vi "uA_Measurement_kit_v2.vi"() -> ()   [LabVIEW 2015]
uses:
  Range_Shunt_selector.ctl
  <vilib>/Waveform/WDTFileIO.llb/ Write Waveform to File.vi
  <vilib>/Waveform/WDTFileIO.llb/Read Waveform from File.vi
  <vilib>/Utility/config.llb/Write Key (I32).vi
  <vilib>/Utility/config.llb/Write Key (Boolean).vi
  <vilib>/Utility/config.llb/Read Key (I32).vi
  <vilib>/Utility/config.llb/Read Key (Boolean).vi
  <vilib>/measure/madcrms.llb/Basic Averaged DC-RMS for 1 Chan.vi
  <resource>/objmgr/daqmx.rc
  <vilib>/Utility/config.llb/NI_LVConfig.lvlib
  <vilib>/measure/NI_MAPro.lvlib
panel:
  out "error out 3":errorcluster
  out "PhysicalChanName":tag
  out "DEV SN":u64 format="%.0x"
  out "mARange":dbl
  out "Boolean":bool
  out "DevSerialNum":u32
  in  "uA_bank0":dbl=1.5 format="%#_13g"
  out "Task out":refnum<k21>="Stop"
  out "Sample rate":dbl=20000.0 format="%#_13g"
  out "Clear":bool=TRUE
  out "Ver":string
  out "seconds since 1Jan1904":timestamp
  in  "Tab Control":enum32{"Current Tracking", "Logging"}(tab)
  out "out_range":bool
  in  "Save setting":bool
  out "PW_Source":bool
  out "EX_IN_INdicator":bool
  in  "LDO":string
  out "Lable.Unit_VOl_MA_UA":string
  in  "Ext PW Vol Monitor":bool
  out "POWER ON_OFF":bool
  out "vbat_lb":dbl format="%#_4f"
  in  "bypass Shunt":bool
  in  "Internal PW":bool
  in  "USB":tag="Dev1"
  out "schematic":bool
  in  "Save":bool
  in  "Load":bool
  out "uA_bank1":dbl
  in  "Calib":bool
  in  "Power ON/OFF":bool
  in  "Profile":enum16{"SAM", "DIANA", "Hi-POWER", "Other..."}(ring)
  in  "Take Picture":bool
  in  "Orginal":bool
  in  "Clear Graph":bool
  in  "ZOOM M1M2":bool
  in  "ZOOM -":bool
  in  "ZOOM +":bool
  in  "stop":bool
  out "Vbat":dbl format="%#.3f"
  in  "Measure":bool
  in  "Range - Shunts":T1
  out "PW_Internal_Source":dbl
  out "Min":dbl
  out "Max":dbl
  out "Delta(s)":sgl
  in  "Center":bool
  out "Avg":dbl
  out "Waveform_main":waveform(sgl)(graph)
  out "Waveform_sub":waveform(dbl)(graph)
  out "Average (uA)":dbl format="%#_6f"
  in  "Vout  - Vbat profile":enum16{"3.8VDC", "2.9VDC", "By Pass", "4.0VDC"}(ring)=enum."2.9VDC" caption="Vout  - Vbat"
  # "µPower kit V2.2"
  # "Vbat"
  # "Vdut- Vbat"
  # "DUT"
  # "Rs"
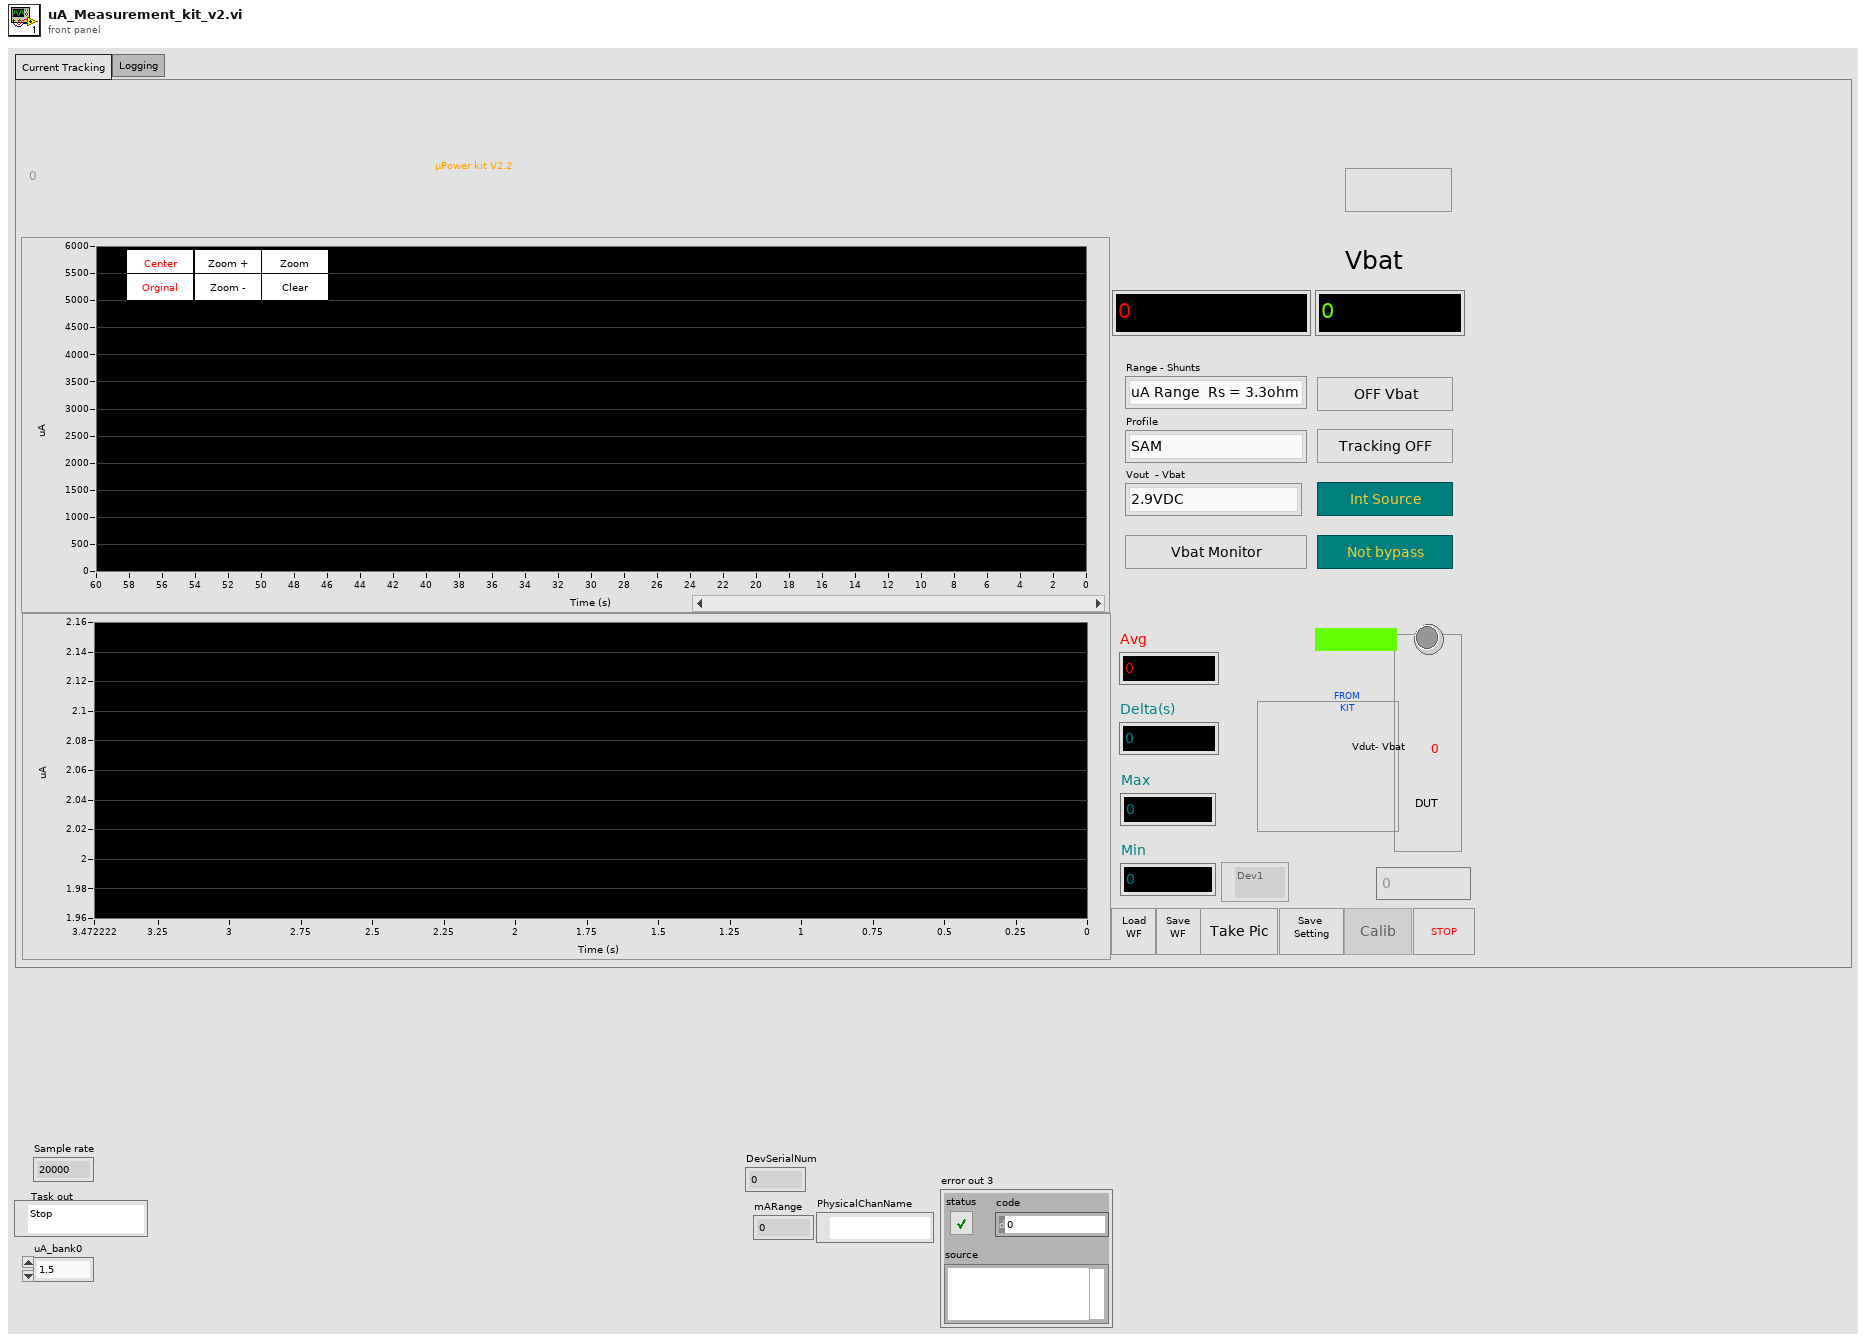
[diagram p1: front panel]
types:
  T1 = typedef "Range_Shunt_selector.ctl" = enum16{"uA Range  Rs = 3.3ohm", "mA Range Rs = 3.3ohm", "mA Range Rs = 1ohm", "mA Range Rs = 1ohm - X2"}
  T2 = enum8{"Enabled", "Disabled", "Disabled and Grayed Out"}
  T3 = typedef "NI_LVConfig.lvlib/Config Data RefNum.ctl" = refnum<k1>
  T4 = enum16{"Internal PW Source", "External PW Source"}
  T5 = enum16{"Turn On bypass - Off Shunt", "Turn Off bypass - On Shunt"}
  T6 = typedef "LVCursorListTypeDef.ctl" = cluster{"Name":string, "Color":u32, "Style":u8, "Point Style":u8, "Name Visible":bool, "Allow Drag":bool, "Cursor Mode":u32, "Plot":i32, "Index":i32, "Position":cluster{"X":dbl, "Y":dbl}, "X Scale":u32, "Y Scale":u32, "Watch Plots":i32[], "Watch All Plots":bool, "Plot Area":i32, "Label Offset":cluster{"X":dbl, "Y":dbl}}[]
  T7 = typedef "imagedata.ctl" = cluster{"image type":i32, "image depth":i32, "image":u8[], "mask":u8[], "colors":u32[], "Rectangle":cluster{"left":i16, "top":i16, "right":i16, "bottom":i16}}
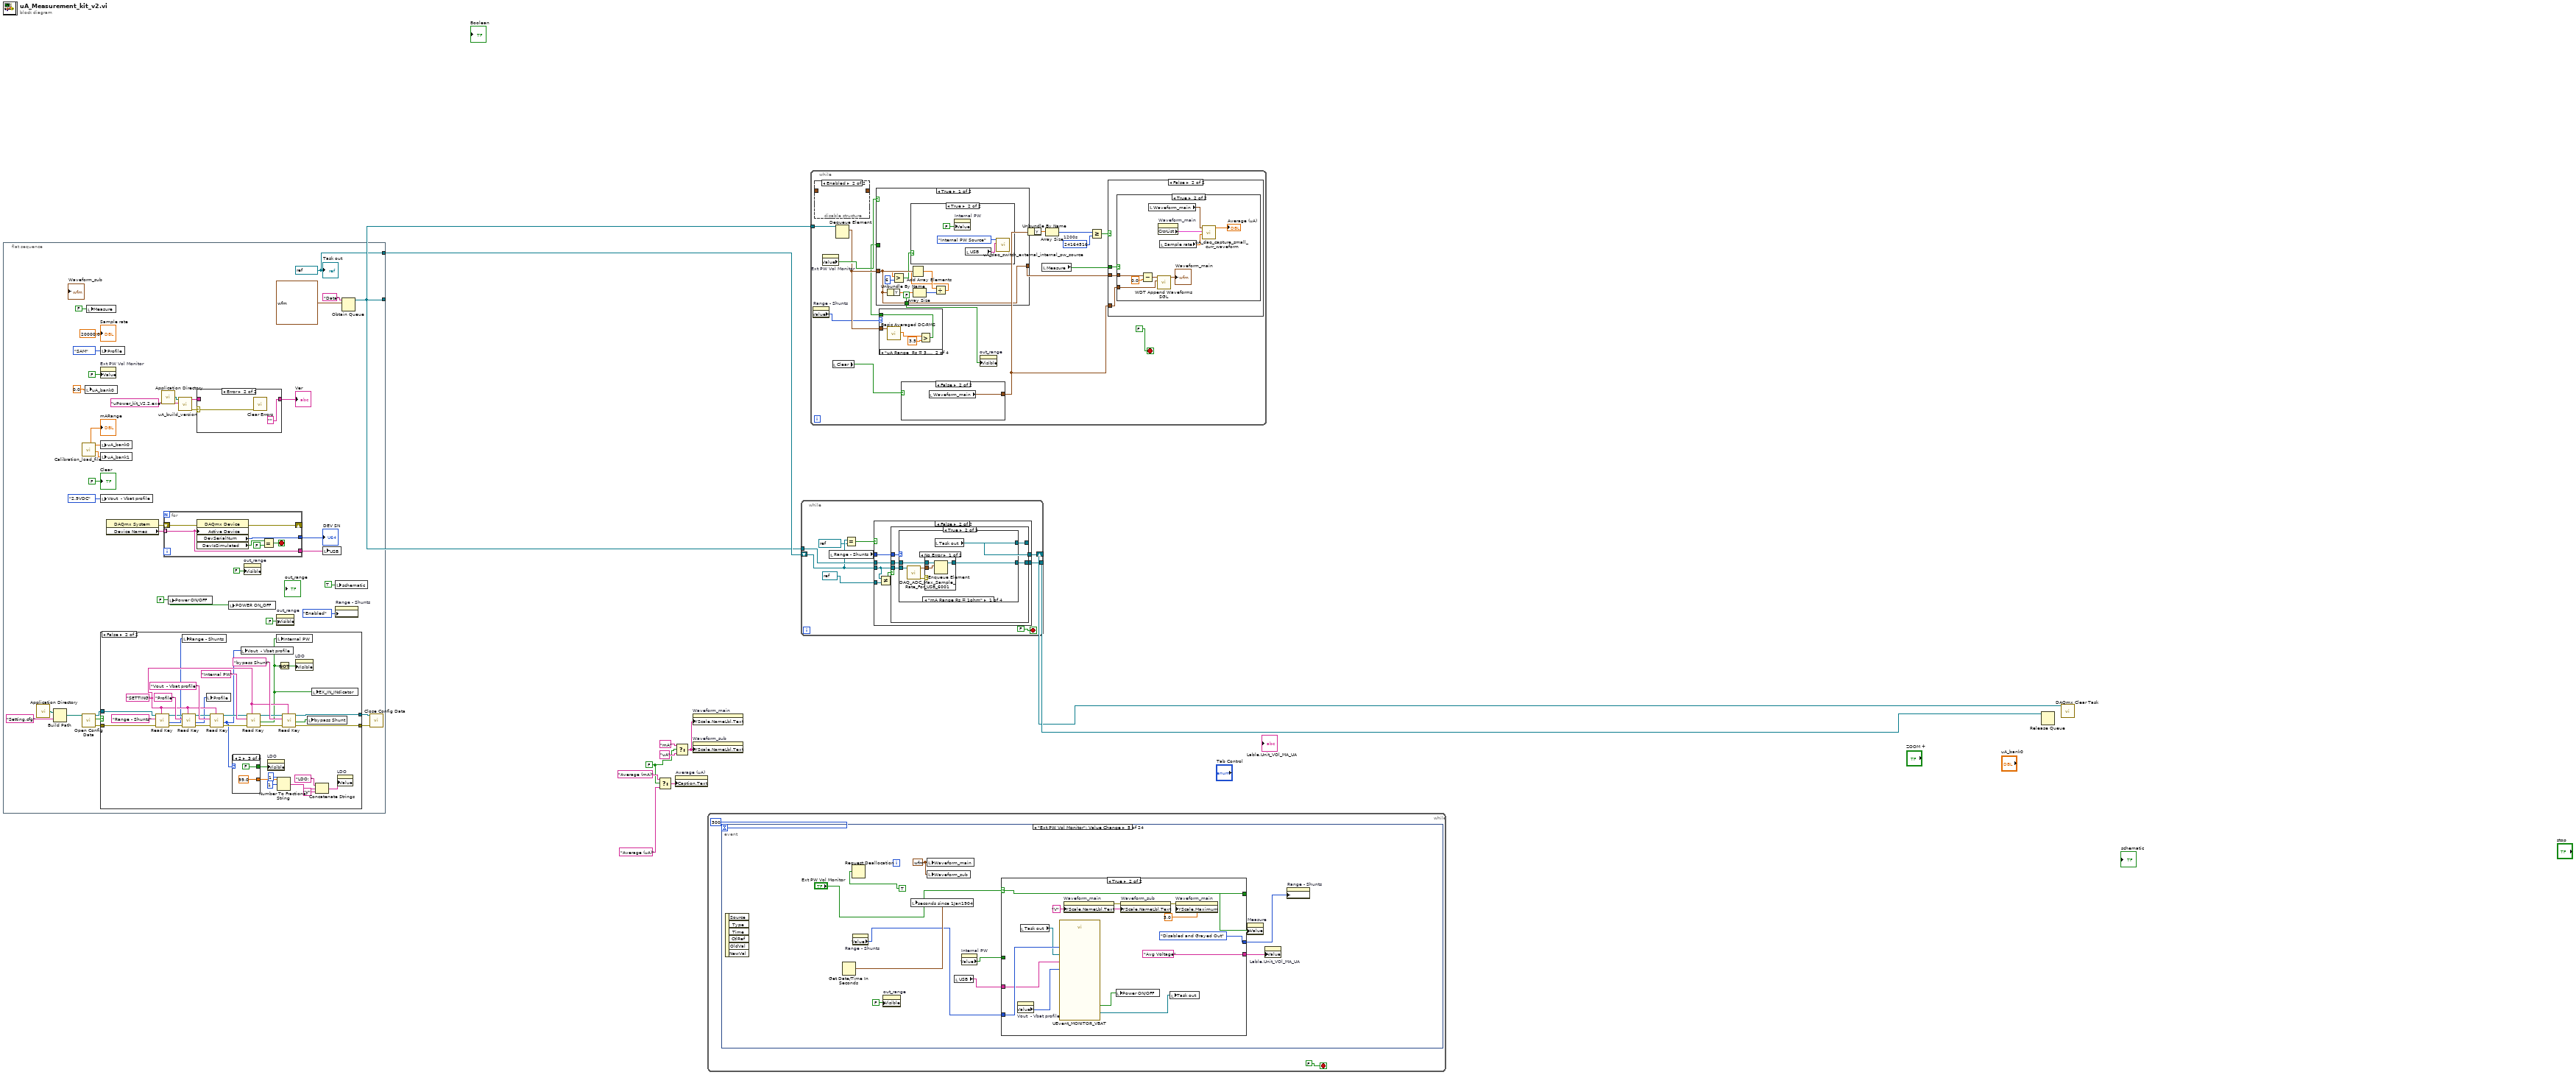
[diagram p0: block diagram]
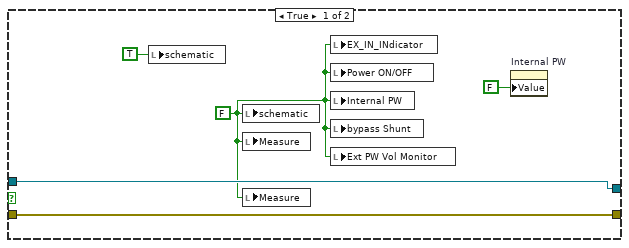
[diagram p2: hidden frame]
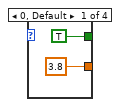
[diagram p3: hidden frame]
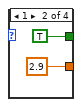
[diagram p4: hidden frame]
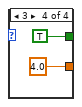
[diagram p5: hidden frame]
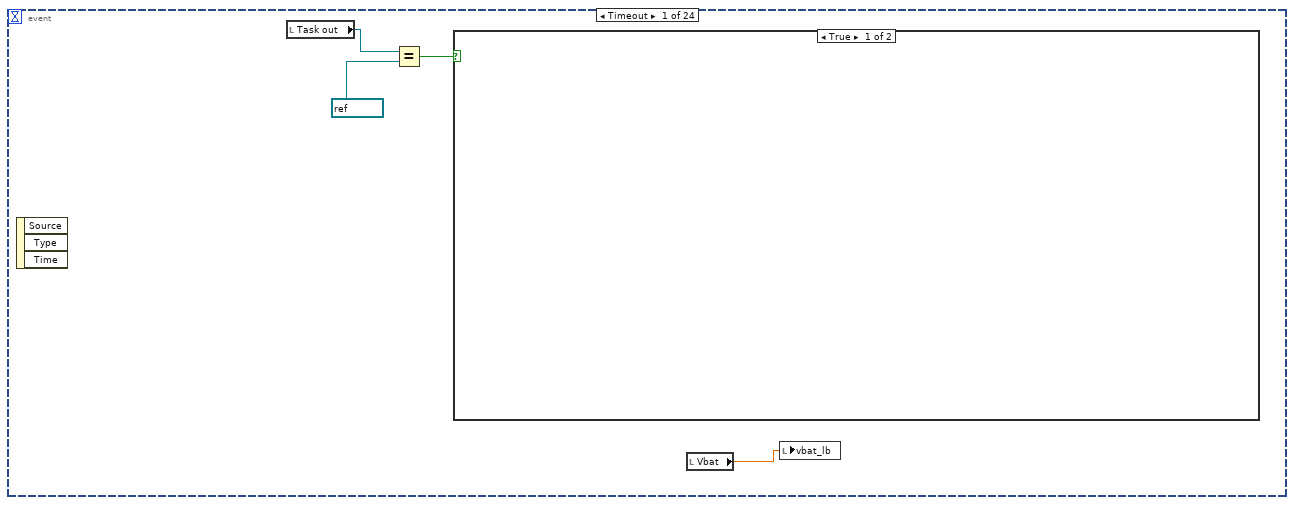
[diagram p7: hidden frame]
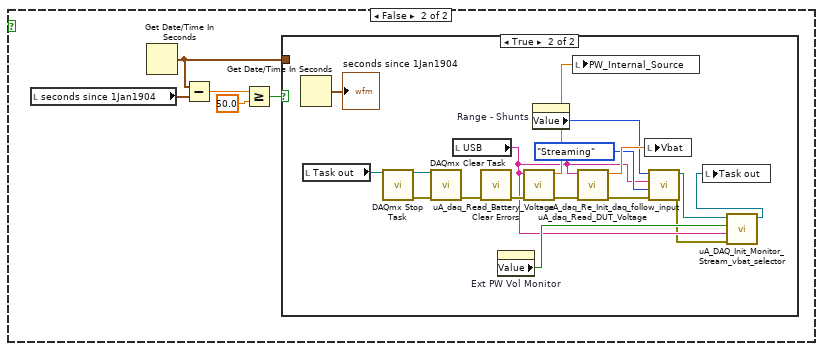
[diagram p8: hidden frame]
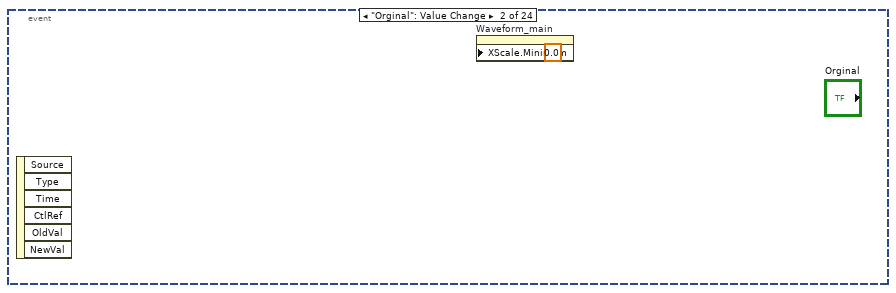
[diagram p10: hidden frame]
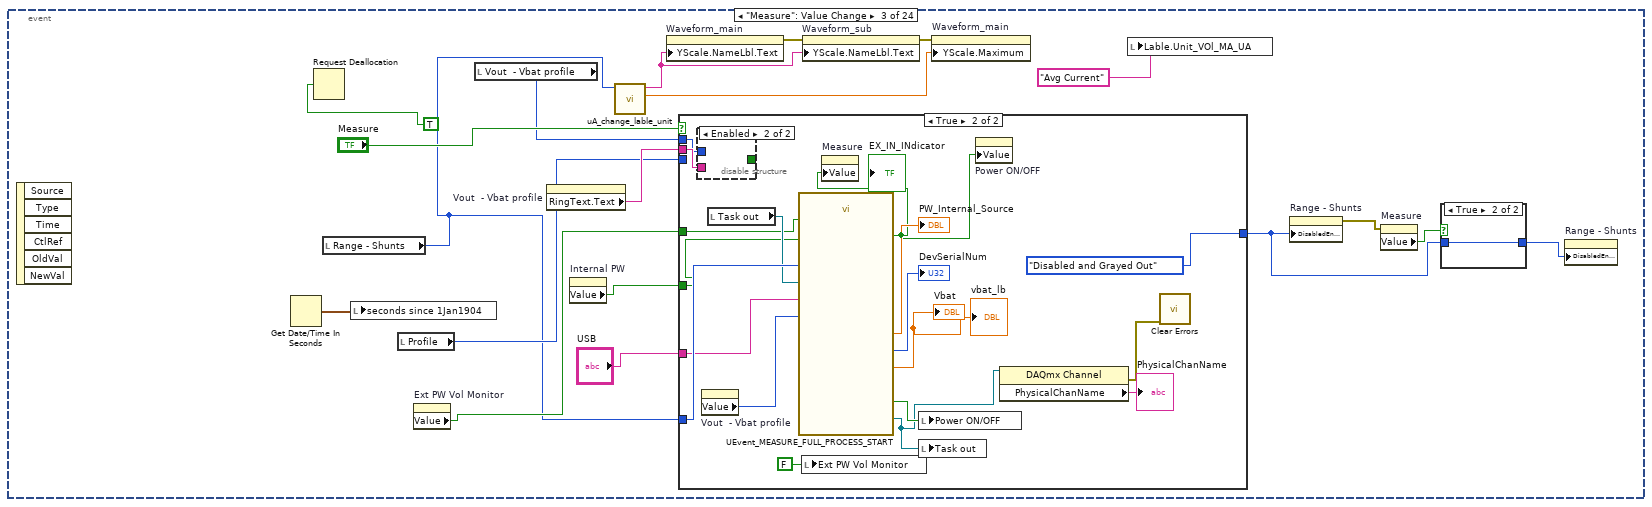
[diagram p11: hidden frame]
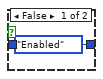
[diagram p12: hidden frame]
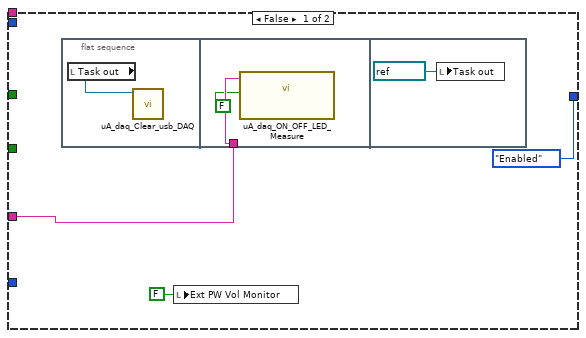
[diagram p13: hidden frame]
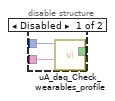
[diagram p14: hidden frame]
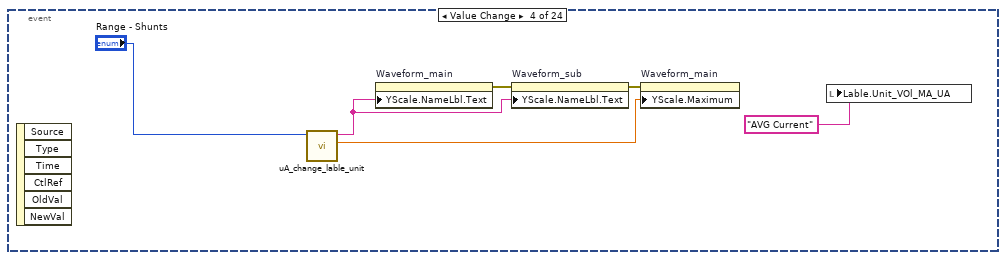
[diagram p15: hidden frame]
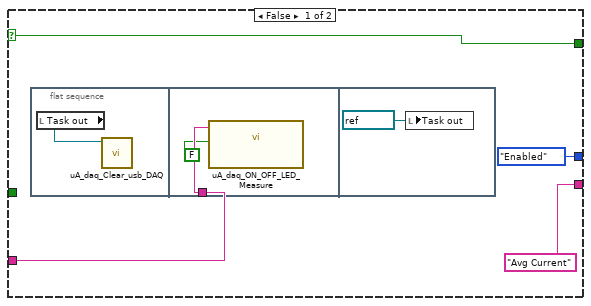
[diagram p16: hidden frame]
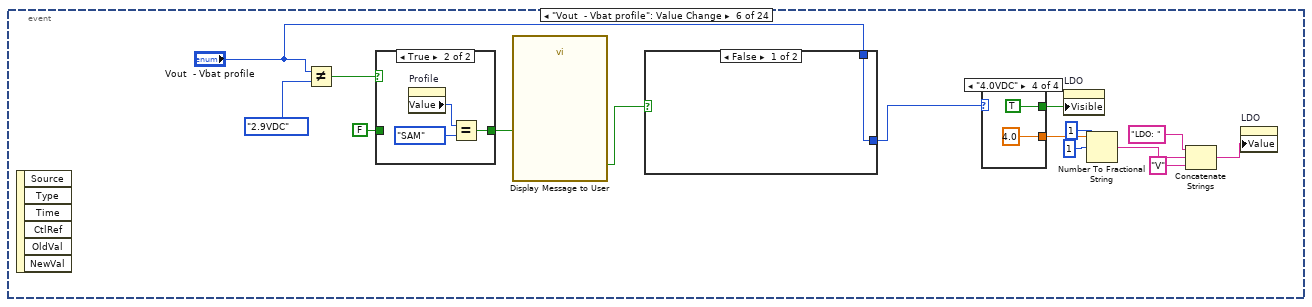
[diagram p17: hidden frame]
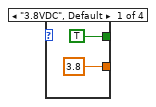
[diagram p18: hidden frame]
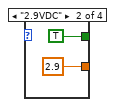
[diagram p19: hidden frame]
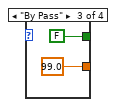
[diagram p20: hidden frame]
diagram:
  w1 = FALSE ("s")
  n1 = flat-sequence {
    tunnel: [w40] -> w3
    tunnel: [w43] -> w2
    frame #0 {
      w16 = FALSE ("Power ON/OFF")
      w40 = refnum<k21> "Stop" ("task out")
      n2 = call <vilib>:"Application Directory.vi"() -> ("Application Directory"=w23:path)
      n3 = Build Path(base path=w23, name or relative path="Setting.cfg") -> (appended path=w21:path)
      n4 = call "Calibration_load_file.vi"() -> ("uABank1"=w33:dbl, "uABank0"=w34:dbl, "mARange"=→"mARange":dbl)  [unwired: 8 in, 1 out]
      n5 = call <vilib>:"Open Config Data.vi"("configuration file path"=w21) -> ("error out"=w17:errorcluster, "file created?"=w24:bool, "refnum"=w20:T3)  [unwired: 8 in]
      n6 = local write "uA_bank0"(0.0 ("uA_calib_0")) -> ()
      n7 = local write "Measure"(FALSE ("Measure")) -> ()
      n8 = local write "Profile"(enum16{"SAM", "DIANA", "Hi-POWER", "Other..."}."SAM" ("Profile")) -> ()
      n9 = property on="Ext PW Vol Monitor" class="Bool (strict)"("Value"=FALSE ("Record uA & Vbat")) -> ()  [unwired: 2 in, 2 out]
      n10 = local write "uA_bank0"(w34) -> ()
      n11 = local write "uA_bank1"(w33) -> ()
      n12 = local write "Vout  - Vbat profile"(enum16{"3.8VDC", "2.9VDC", "By Pass", "4.0VDC"}."2.9VDC" ("Vout  - Vbat profile")) -> ()
      n13 = case shown="False" w24 {
        tunnel: w17 -> [w52 w84]
        tunnel: [w52 w79] -> w18
        tunnel: [w51 w78] -> w19
        tunnel: w20 -> [w51 w67]
        frame True {
          w50 = FALSE ("Measure")
          n14 = local write "schematic"(TRUE ("schematic")) -> ()
          n15 = local write "schematic"(w50) -> ()
          n16 = local write "Measure"(w50) -> ()
          n17 = local write "Measure"(w50) -> ()
          n18 = local write "EX_IN_INdicator"(w50) -> ()
          n19 = local write "Power ON/OFF"(w50) -> ()
          n20 = local write "Internal PW"(w50) -> ()
          n21 = local write "bypass Shunt"(w50) -> ()
          n22 = local write "Ext PW Vol Monitor"(w50) -> ()
          n23 = property on="Internal PW" class="Bool (strict)"("Value"=FALSE ("Internal PW")) -> ()  [unwired: 2 in, 2 out]
        }
        frame False {
          w68 = "SETTING" ("section")
          n24 = call-poly <vilib>:"Read Key.vi"("section"=w68, "error in (no error)"=w84, "key"="Range - Shunts", "refnum"=w67) -> ("error out"=w83:errorcluster, "value"=w66:i32, "refnum out"=w70:T3)  [unwired: 4 in, 1 out]
          n25 = local write "Range - Shunts"(w66) -> ()
          n26 = call-poly <vilib>:"Read Key.vi"("section"=w68, "error in (no error)"=w83, "key"="Profile", "refnum"=w70) -> ("error out"=w82:errorcluster, "value"=w65:i32, "refnum out"=w69:T3)  [unwired: 4 in, 1 out]
          n27 = local write "Profile"(w65) -> ()
          n28 = call-poly <vilib>:"Read Key.vi"("section"=w68, "error in (no error)"=w82, "key"="Vout  - Vbat profile", "refnum"=w69) -> ("error out"=w81:errorcluster, "value"=w53:i32, "refnum out"=w71:T3)  [unwired: 4 in, 1 out]
          n29 = case shown="2" w53 {
            tunnel: [3.8 2.9 99.0 4.0] -> w58
            tunnel: [TRUE ("Visible") TRUE ("Visible") FALSE ("Visible") TRUE ("Visible")] -> w59
            frame 0, Default {
            }
            frame 1 {
            }
            frame 2 {
            }
            frame 3 {
            }
          }
          n30 = local write "Vout  - Vbat profile"(w53) -> ()
          n31 = call-poly <vilib>:"Read Key.vi"("section"=w68, "error in (no error)"=w81, "key"="Internal PW", "refnum"=w71) -> ("error out"=w80:errorcluster, "value"=w62:bool, "refnum out"=w72:T3)  [unwired: 4 in, 1 out]
          n32 = property on="LDO" class="Str"("Visible"=w59) -> ()  [unwired: 2 in, 2 out]
          n33 = local write "Internal PW"(w62) -> ()
          n34 = Number To Fractional String(number=w58, width (-)=i16 1, precision (6)=i16 1) -> (F-format string=w55:string)  [unwired: 1 in]
          n35 = Not(x=w62) -> (.not. x?=w63:bool)
          n36 = call-poly <vilib>:"Read Key.vi"("section"=w68, "error in (no error)"=w80, "key"="bypass Shunt", "refnum"=w72) -> ("error out"=w79:errorcluster, "value"=w64:bool, "refnum out"=w78:T3)  [unwired: 4 in, 1 out]
          n37 = property on="LDO" class="Str"("Visible"=w63) -> ()  [unwired: 2 in, 2 out]
          n38 = local write "bypass Shunt"(w64) -> ()
          n39 = local write "EX_IN_INdicator"(w62) -> ()
          n40 = Concatenate Strings("LDO: " ("string"), w55, "V" ("string")) -> (w54:string)
          n41 = property on="LDO" class="Str"("Value"=w54) -> ()  [unwired: 2 in, 2 out]
        }
      }
      n42 = property class="DAQmx System"() -> (error out=w31:errorcluster, "Device Names"=w32:tag[])  [unwired: 2 in, 1 out]
      n43 = call <vilib>:"Application Directory.vi"() -> ("Application Directory"=w42:path)
      n44 = for {
        tunnel: w32 -> [w94] mode=indexing
        shift-right: [w98] -> _
        shift-left: w31 -> [w99]
        tunnel: [w94] -> w30
        tunnel: [w93] -> w28
        stop <- w95 stop-if-true
        n45 = property class="DAQmx Device"(error in=w99, "Active Device"=w94) -> (error out=w98:errorcluster, "DevSerialNum"=w93:u32, "DevIsSimulated"=w97:bool)  [unwired: 1 in, 1 out]
        n46 = Equal?(x=w97, y=FALSE) -> (x = y?=w95:bool)
      }
      "DEV SN" <- w28
      n47 = local write "Power ON/OFF"(w16) -> ()
      n48 = call "uA_build_version.vi"("name or relative path"="uPower_kit_V2.2.exe", "path"=w42) -> ("error out"=w39:errorcluster, "FileVersion"=w38:string)  [unwired: 7 in, 1 out]
      n49 = case shown="Error" w39 {
        selector: w39 -> [_ w102]
        tunnel: w38 -> [w100 _]
        tunnel: [w100 "" ("FileVersion")] -> w37
        frame No Error {
        }
        frame Error {
          n50 = call <vilib>:"Clear Errors.vi"("error in (no error)"=w102) -> ()  [unwired: 5 in, 2 out]
        }
      }
      "Ver" <- w37
      n51 = local write "POWER ON_OFF"(w16) -> ()
      n52 = property on="out_range" class="Bool (strict)"("Visible"=FALSE) -> ()  [unwired: 2 in, 2 out]
      n53 = property on="out_range" class="Bool (strict)"("Visible"=FALSE) -> ()  [unwired: 2 in, 2 out]
      n54 = local write "USB"(w30) -> ()
      n55 = local write "schematic"(TRUE ("schematic")) -> ()
      n56 = property on="Range - Shunts" class="Enum (strict)"("DisabledEnum"=T2."Enabled" ("Disabled")) -> ()  [unwired: 2 in, 2 out]
      n57 = Obtain Queue(name (unnamed)="Data", element data type=waveform(sgl) {"t0"=timestamp(0 s since 1904-01-01), "dt"=1.0, "Y"=[]} ("Waveform Chart 2")) -> (queue out=w43:refnum<queue>)  [unwired: 3 in, 2 out]
      n58 = call <vilib>:"Close Config Data.vi"("error in (no error)"=w18, "refnum"=w19) -> ()  [unwired: 8 in, 2 out]
      "Clear" <- FALSE ("Clear")
      "Sample rate" <- 20000.0 ("Sample rate")
      "Task out" <- w40
    }
  }
  n59 = Select(t="Average (mA)" ("Caption.Text"), s=w1, f="Average (uA)" ("Caption.Text")) -> (s? t:f=w5:string)
  n60 = property on="Average (uA)" class="DigNum (strict)"("Caption.Text"=w5) -> ()  [unwired: 2 in, 2 out]
  n61 = Select(t="mA" ("Caption.Text"), s=w1, f="uA" ("Caption.Text")) -> (s? t:f=w6:string)
  n62 = property on="Waveform_main" class="WFGraph (strict)"("YScale.NameLbl.Text"=w6) -> ()  [unwired: 2 in, 2 out]
  n63 = property on="Waveform_sub" class="WFGraph (strict)"("YScale.NameLbl.Text"=w6) -> ()  [unwired: 2 in, 2 out]
  n64 = while {
    stop <- FALSE stop-if-true
    n65 = event shown="[4] \"Ext PW Vol Monitor\": Value Change" {
      selector: _ -> [_ _ _ _ _ _ _ _ _ _ _ _ _ _ _ _ _ _ _ _ _ _ _ _]
      dyn-events: _ -> [_ _ _ _ _ _ _ _ _ _ _ _ _ _ _ _ _ _ _ _ _ _ _ _]
      timeout: 300 -> [_ _ _ _ _ _ _ _ _ _ _ _ _ _ _ _ _ _ _ _ _ _ _ _]
      event Timeout {
        n66 = event-data() -> ()  [unwired: 1 in, 3 out]
        n67 = local read "Task out"() -> (w106:refnum<k21>)
        n68 = Equal?(x=w106, y=refnum<k21> "Stop") -> (x = y?=w107:bool)
        n69 = case shown="True" w107 {
          frame True {
          }
          frame False {
            n70 = local read "seconds since 1Jan1904"() -> (w109:timestamp)
            n71 = Get Date/Time In Seconds() -> (seconds since 1Jan1904=w110:timestamp)
            n72 = Subtract(x=w110, y=w109) -> (x-y=w113:dbl)
            n73 = Greater Or Equal?(x=w113, y=50.0) -> (x >= y?=w111:bool)
            n74 = case shown="True" w111 {
              tunnel: w110 -> [_ _]
              frame False {
              }
              frame True {
                n75 = Get Date/Time In Seconds() -> (seconds since 1Jan1904=→"seconds since 1Jan1904":timestamp)
                n76 = local read "Task out"() -> (w127:refnum<k21>)
                n77 = call <vilib>:"DAQmx Stop Task.vi"("task/channels in"=w127) -> ("task out"=w126:refnum<k21>, "error out"=w129:errorcluster)  [unwired: 13 in]
                n78 = call <vilib>:"DAQmx Clear Task.vi"("task in"=w126, "error in"=w129) -> ("error out"=w128:errorcluster)  [unwired: 13 in]
                n79 = local read "USB"() -> (w115:tag)
                n80 = call <vilib>:"Clear Errors.vi"("error in (no error)"=w128) -> ("error out"=w125:errorcluster)  [unwired: 5 in, 1 out]
                n81 = property on="Ext PW Vol Monitor" class="Bool (strict)"() -> ("Value"=w116:bool)  [unwired: 2 in, 2 out]
                n82 = call "uA_daq_Read_Battery_Voltage.vi"("error in"=w125, "USB DAQ"=w115) -> ("error out"=w122:errorcluster, "Battery_Voltage"=w124:dbl)  [unwired: 8 in]
                n83 = property on="Range - Shunts" class="Enum (strict)"() -> ("Value"=w121:T1)  [unwired: 2 in, 2 out]
                n84 = local write "PW_Internal_Source"(w124) -> ()
                n85 = call "uA_daq_Read_DUT_Voltage.vi"("error in"=w122, "USB DAQ"=w115) -> ("error out"=w120:errorcluster, "DUT_Voltage"=w123:dbl)  [unwired: 8 in]
                n86 = local write "Vbat"(w123) -> ()
                n87 = call "uA_daq_Re_Init_daq_follow_input.vi"("error in (no error)"=w120, "Acquire Mode"=enum16{"Streaming", "Read All", "Stop"}."Streaming", "USB"=w115, "Range_shunt"=w121) -> ("error out"=w114:errorcluster, "Refnum out"=w118:refnum<k21>)  [unwired: 6 in]
                n88 = call "uA_DAQ_Init_Monitor_Stream_vbat_selector.vi"("error in (no error)"=w114, "USB"=w115, "Ext PW Vol Monitor"=w116, "Refnum in"=w118) -> ("Refnum out"=w117:refnum<k21>)  [unwired: 6 in, 1 out]
                n89 = local write "Task out"(w117) -> ()
              }
            }
          }
        }
        n90 = local read "Vbat"() -> (w105:dbl)
        n91 = local write "vbat_lb"(w105) -> ()
      }
      event "Orginal": Value Change {
        n92 = event-data() -> ()  [unwired: 1 in, 6 out]
        n93 = property on="Waveform_main" class="WFGraph (strict)"("XScale.Minimum"=0.0 ("X Scale.Range:Minimum")) -> ()  [unwired: 2 in, 2 out]
      }
      event "Measure": Value Change {
        n94 = event-data() -> ()  [unwired: 1 in, 6 out]
        n95 = Get Date/Time In Seconds() -> (seconds since 1Jan1904=w149:timestamp)
        n96 = Request Deallocation(TRUE ("flag")) -> ()
        n97 = local read "Range - Shunts"() -> (w136:T1)
        n98 = local write "seconds since 1Jan1904"(w149) -> ()
        n99 = local read "Profile"() -> (w145:enum16{"SAM", "DIANA", "Hi-POWER", "Other..."})
        n100 = property on="Ext PW Vol Monitor" class="Bool (strict)"() -> ("Value"=w138:bool)  [unwired: 2 in, 2 out]
        n101 = local read "Vout  - Vbat profile"() -> (w146:enum16{"3.8VDC", "2.9VDC", "By Pass", "4.0VDC"})
        n102 = property on="Vout  - Vbat profile" class="Enum (strict)"() -> ("RingText.Text"=w147:string)  [unwired: 2 in, 2 out]
        n103 = property on="Internal PW" class="Bool (strict)"() -> ("Value"=w140:bool)  [unwired: 2 in, 2 out]
        n104 = call "uA_change_lable_unit.vi"("Range - Shunts"=w136) -> ("Y_scale"=w142:dbl, "unit"=w141:string)  [unwired: 8 in, 1 out]
        n105 = property on="Waveform_main" class="WFGraph (strict)"("YScale.NameLbl.Text"=w141) -> (error out=w144:errorcluster)  [unwired: 2 in, 1 out]
        n106 = case shown="True" "Measure" {
          tunnel: w147 -> [_ w177]
          tunnel: w146 -> [_ w176]
          tunnel: w145 -> [_ _]
          tunnel: w136 -> [_ w172]
          tunnel: w140 -> [_ w168]
          tunnel: "USB" -> [w154 w166]
          tunnel: w138 -> [_ w163]
          tunnel: [T2."Enabled" ("Disabled") T2."Disabled and Grayed Out" ("Disabled")] -> w132
          frame False {
            n107 = flat-sequence {
              tunnel: w154 -> [w158]
              frame #0 {
                n108 = local read "Task out"() -> (w156:refnum<k21>)
                n109 = call "uA_daq_Clear_usb_DAQ.vi"("Refnum in"=w156) -> ()  [unwired: 11 in]
              }
              frame #1 {
                n110 = call "uA_daq_ON_OFF_LED_Measure.vi"("LED_meas"=FALSE ("Boolean"), "USB"=w158) -> ()  [unwired: 9 in, 1 out]
              }
              frame #2 {
                n111 = local write "Task out"(refnum<k21> "Stop" ("Refnum out")) -> ()
              }
            }
            n112 = local write "Ext PW Vol Monitor"(FALSE ("Ext PW Vol Monitor")) -> ()
          }
          frame True {
            n113 = disable-structure shown="Enabled" {
              disable-tunnel: w177 -> [w180 _]
              disable-tunnel: w176 -> [w179 _]
              disable-tunnel: [w178 _] -> _
              frame Disabled {
                n114 = call "uA_daq_Check_wearables_profile.vi"("VDUT"=w180, "DUT Voltage Selector"=w179) -> ("Profile"=w178:bool)  [unwired: 8 in, 1 out]
              }
              frame Enabled {
              }
            }
            n115 = property on="Vout  - Vbat profile" class="Enum (strict)"() -> ("Value"=w169:enum16{"3.8VDC", "2.9VDC", "By Pass", "4.0VDC"})  [unwired: 2 in, 2 out]
            n116 = local read "Task out"() -> (w171:refnum<k21>)
            n117 = call "UEvent_MEASURE_FULL_PROCESS_START.vi"("Refnum in"=w171, "Range - Shunts"=w172, "Ext PW Vol Monitor"=w163, "USB"=w166, "Internal/external Power"=w168, "Vout  - Vbat profile"=w169) -> ("DevSerialNum"=→"DevSerialNum":u32, "Power ON/OFF"=w174:bool, "Refnum out"=w165:refnum<k21>, "Battery_Voltage"=→"PW_Internal_Source":dbl, "DUT_Voltage"=→"Vbat" →"vbat_lb":dbl, "Measure indicator"=w167:bool)  [unwired: 3 in, 1 out]
            n118 = local write "Ext PW Vol Monitor"(FALSE ("Ext PW Vol Monitor")) -> ()
            n119 = property on="Measure" class="Bool (strict)"("Value"=w167) -> ()  [unwired: 2 in, 2 out]
            n120 = local write "Power ON/OFF"(w174) -> ()
            n121 = local write "Task out"(w165) -> ()
            n122 = property on="Power ON/OFF" class="Bool (strict)"("Value"=w167) -> ()  [unwired: 2 in, 2 out]
            n123 = property class="DAQmx Channel"(reference=w165) -> (error out=w162:errorcluster, "PhysicalChanName"=→"PhysicalChanName":tag)  [unwired: 1 in, 1 out]
            n124 = call <vilib>:"Clear Errors.vi"("error in (no error)"=w162) -> ()  [unwired: 5 in, 2 out]
          }
        }
        n125 = property on="Waveform_sub" class="WFGraph (strict)"(error in=w144, "YScale.NameLbl.Text"=w141) -> (error out=w143:errorcluster)  [unwired: 1 in, 1 out]
        n126 = property on="Waveform_main" class="WFGraph (strict)"(error in=w143, "YScale.Maximum"=w142) -> ()  [unwired: 1 in, 2 out]
        n127 = local write "Lable.Unit_VOl_MA_UA"("Avg Current" ("Lable.Unit_VOl_MA_UA")) -> ()
        n128 = property on="Range - Shunts" class="Enum (strict)"("DisabledEnum"=w132) -> (error out=w135:errorcluster)  [unwired: 2 in, 1 out]
        n129 = property on="Measure" class="Bool (strict)"(error in=w135) -> ("Value"=w134:bool)  [unwired: 1 in, 2 out]
        n130 = case shown="True" w134 {
          tunnel: [T2."Enabled" ("Disabled") w152] -> w133
          tunnel: w132 -> [_ w152]
          frame False {
          }
          frame True {
          }
        }
        n131 = property on="Range - Shunts" class="Enum (strict)"("DisabledEnum"=w133) -> ()  [unwired: 2 in, 2 out]
      }
      event Value Change {
        n132 = event-data() -> ()  [unwired: 1 in, 6 out]
        n133 = call "uA_change_lable_unit.vi"("Range - Shunts"="Range - Shunts") -> ("Y_scale"=w184:dbl, "unit"=w183:string)  [unwired: 8 in, 1 out]
        n134 = property on="Waveform_main" class="WFGraph (strict)"("YScale.NameLbl.Text"=w183) -> (error out=w186:errorcluster)  [unwired: 2 in, 1 out]
        n135 = property on="Waveform_sub" class="WFGraph (strict)"(error in=w186, "YScale.NameLbl.Text"=w183) -> (error out=w185:errorcluster)  [unwired: 1 in, 1 out]
        n136 = property on="Waveform_main" class="WFGraph (strict)"(error in=w185, "YScale.Maximum"=w184) -> ()  [unwired: 1 in, 2 out]
        n137 = local write "Lable.Unit_VOl_MA_UA"("AVG Current" ("Lable.Unit_VOl_MA_UA")) -> ()
      }
      event "Ext PW Vol Monitor": Value Change {
        w189 = waveform(sgl) {"t0"=timestamp(0 s since 1904-01-01), "dt"=1.0, "Y"=[]} ("Waveform_main")
        n138 = event-data() -> ()  [unwired: 1 in, 6 out]
        n139 = Get Date/Time In Seconds() -> (seconds since 1Jan1904=w196:timestamp)
        n140 = Request Deallocation(TRUE ("flag")) -> ()
        n141 = property on="Range - Shunts" class="Enum (strict)"() -> ("Value"=w193:T1)  [unwired: 2 in, 2 out]
        n142 = property on="out_range" class="Bool (strict)"("Visible"=FALSE) -> ()  [unwired: 2 in, 2 out]
        n143 = local write "seconds since 1Jan1904"(w196) -> ()
        n144 = local write "Waveform_main"(w189) -> ()
        n145 = local write "Waveform_sub"(w189) -> ()
        n146 = local read "USB"() -> (w192:tag)
        n147 = property on="Internal PW" class="Bool (strict)"() -> ("Value"=w195:bool)  [unwired: 2 in, 2 out]
        n148 = case shown="True" "Ext PW Vol Monitor" {
          selector: "Ext PW Vol Monitor" -> [w200 w213]
          tunnel: w193 -> [_ w217]
          tunnel: w195 -> [_ _]
          tunnel: w192 -> [w201 w214]
          tunnel: [w200 w213] -> w191
          tunnel: ["Avg Current" ("Lable.Unit_VOl_MA_UA") "Avg Voltage" ("Lable.Unit_VOl_MA_UA")] -> w190
          tunnel: [T2."Enabled" ("Disabled") T2."Disabled and Grayed Out" ("Disabled")] -> w188
          frame False {
            n149 = flat-sequence {
              tunnel: w201 -> [w204]
              frame #0 {
                n150 = local read "Task out"() -> (w202:refnum<k21>)
                n151 = call "uA_daq_Clear_usb_DAQ.vi"("Refnum in"=w202) -> ()  [unwired: 11 in]
              }
              frame #1 {
                n152 = call "uA_daq_ON_OFF_LED_Measure.vi"("LED_meas"=FALSE ("Boolean"), "USB"=w204) -> ()  [unwired: 9 in, 1 out]
              }
              frame #2 {
                n153 = local write "Task out"(refnum<k21> "Stop" ("Refnum out")) -> ()
              }
            }
          }
          frame True {
            w212 = "V" ("Y Scale.Name Label.Text")
            n154 = property on="Vout  - Vbat profile" class="Enum (strict)"() -> ("Value"=w215:enum16{"3.8VDC", "2.9VDC", "By Pass", "4.0VDC"})  [unwired: 2 in, 2 out]
            n155 = local read "Task out"() -> (w216:refnum<k21>)
            n156 = call "UEvent_MONITOR_VBAT.vi"("Vout  - Vbat profile"=w215, "USB"=w214, "Range - Shunts"=w217, "Refnum in"=w216) -> ("Refnum out"=w207:refnum<k21>, "Power ON/OFF"=w218:bool)  [unwired: 2 in, 4 out]
            n157 = property on="Waveform_main" class="WFGraph (strict)"("YScale.NameLbl.Text"=w212) -> (error out=w209:errorcluster)  [unwired: 2 in, 1 out]
            n158 = local write "Power ON/OFF"(w218) -> ()
            n159 = property on="Waveform_sub" class="WFGraph (strict)"(error in=w209, "YScale.NameLbl.Text"=w212) -> (error out=w210:errorcluster)  [unwired: 1 in, 1 out]
            n160 = local write "Task out"(w207) -> ()
            n161 = property on="Waveform_main" class="WFGraph (strict)"(error in=w210, "YScale.Maximum"=5.0 ("Y Scale.Range:Maximum")) -> ()  [unwired: 1 in, 2 out]
          }
        }
        n162 = property on="Measure" class="Bool (strict)"("Value"=w191) -> ()  [unwired: 2 in, 2 out]
        n163 = property on="Lable.Unit_VOl_MA_UA" class="Str"("Value"=w190) -> ()  [unwired: 2 in, 2 out]
        n164 = property on="Range - Shunts" class="Enum (strict)"("DisabledEnum"=w188) -> ()  [unwired: 2 in, 2 out]
      }
      event "Vout  - Vbat profile": Value Change {
        n165 = event-data() -> ()  [unwired: 1 in, 6 out]
        n166 = Not Equal?(x="Vout  - Vbat profile", y=enum16{"3.8VDC", "2.9VDC", "By Pass", "4.0VDC"}."2.9VDC" ("Vout  - Vbat profile")) -> (x != y?=w233:bool)
        n167 = case shown="True" w233 {
          tunnel: [w244 w245] -> w231
          tunnel: FALSE -> [w244 _]
          frame False {
          }
          frame True {
            n168 = property on="Profile" class="Enum (strict)"() -> ("Value"=w247:enum16{"SAM", "DIANA", "Hi-POWER", "Other..."})  [unwired: 2 in, 2 out]
            n169 = Equal?(x=w247, y=enum16{"SAM", "DIANA", "Hi-POWER", "Other..."}."SAM" ("Profile")) -> (x = y?=w245:bool)
          }
        }
        n170 = call "Display Message to User"("Enable"=w231) -> ("OK"=w230:bool)  [unwired: 9 in, 1 out]
        n171 = case shown="False" w230 {
          tunnel: [w242 w243] -> w227
          tunnel: "Vout  - Vbat profile" -> [w242 _]
          frame False {
          }
          frame True {
            w243 = enum16{"3.8VDC", "2.9VDC", "By Pass", "4.0VDC"}."2.9VDC" ("Vout  - Vbat profile")
            n172 = property on="Vout  - Vbat profile" class="Enum (strict)"("Value"=w243) -> ()  [unwired: 2 in, 2 out]
          }
        }
        n173 = case shown="\"4.0VDC\"" w227 {
          tunnel: [3.8 2.9 99.0 4.0] -> w222
          tunnel: [TRUE ("Visible") TRUE ("Visible") FALSE ("Visible") TRUE ("Visible")] -> w221
          frame "3.8VDC", Default {
          }
          frame "2.9VDC" {
          }
          frame "By Pass" {
          }
          frame "4.0VDC" {
          }
        }
        n174 = property on="LDO" class="Str"("Visible"=w221) -> ()  [unwired: 2 in, 2 out]
        n175 = Number To Fractional String(number=w222, width (-)=i16 1, precision (6)=i16 1) -> (F-format string=w225:string)  [unwired: 1 in]
        n176 = Concatenate Strings("LDO: " ("string"), w225, "V" ("string")) -> (w226:string)
        n177 = property on="LDO" class="Str"("Value"=w226) -> ()  [unwired: 2 in, 2 out]
      }
      event "Internal PW": Value Change {
        n178 = event-data() -> ()  [unwired: 1 in, 6 out]
        n179 = case shown="True" "Internal PW" {
          tunnel: [T4."Internal PW Source" ("Ex/Int PW") T4."External PW Source" ("Ex/Int PW")] -> w260
          frame False {
            # "Internal power source"
          }
          frame True {
            # "External Power Source"
          }
        }
        n180 = property on="Ext PW Vol Monitor" class="Bool (strict)"() -> ("Value"=w256:bool)  [unwired: 2 in, 2 out]
        n181 = property on="Range - Shunts" class="Enum (strict)"() -> ("Value"=w259:T1)  [unwired: 2 in, 2 out]
        n182 = local read "Task out"() -> (w263:refnum<k21>)
        n183 = local read "USB"() -> (w258:tag)
        n184 = call "UEvent_SET_INTERNAL_EXTERNAL_POWER_SOURCE.vi"("Ex/Int PW"=w260, "Ext PW Vol Monitor"=w256, "USB"=w258, "Value"=w259, "Refnum in"=w263) -> ("External Voltage HIGH"=w255:bool, "Battery_Voltage"=w262:dbl, "DUT_Voltage"=w261:dbl, "Refnum out"=w257:refnum<k21>)  [unwired: 3 in]
        n185 = local read "Measure"() -> (w254:bool)
        n186 = local write "Vbat"(w261) -> ()
        n187 = local write "PW_Internal_Source"(w262) -> ()
        n188 = case shown="False" w254 {
          tunnel: w257 -> [_ w269]
          tunnel: [refnum<k21> "Stop" ("Refnum out") w269] -> w253
          frame False {
          }
          frame True {
          }
        }
        n189 = case shown="True" w255 {
          tunnel: w255 -> [_ w271]
          tunnel: [w270 w271] -> w250
          tunnel: "Internal PW" -> [w270 _]
          frame True {
          }
          frame False {
            n190 = property on="Internal PW" class="Bool (strict)"("Value"=w271) -> ()  [unwired: 2 in, 2 out]
          }
        }
        n191 = local write "Task out"(w253) -> ()
        n192 = local read "Vout  - Vbat profile"() -> (w251:enum16{"3.8VDC", "2.9VDC", "By Pass", "4.0VDC"})
        n193 = Not(x=w250) -> (.not. x?=w248:bool)
        n194 = case shown="\"By Pass\"" w251 {
          tunnel: w248 -> [w264 w265 _ w267]
          tunnel: [w264 w265 FALSE w267] -> w249
          frame "3.8VDC", Default {
          }
          frame "2.9VDC" {
          }
          frame "By Pass" {
          }
          frame "4.0VDC" {
          }
        }
        n195 = property on="LDO" class="Str"("Visible"=w249) -> ()  [unwired: 2 in, 2 out]
        n196 = local write "EX_IN_INdicator"(w250) -> ()
        "PW_Source" <- "Internal PW"
      }
      event "bypass Shunt": Value Change {
        n197 = event-data() -> ()  [unwired: 1 in, 6 out]
        n198 = Not(x="bypass Shunt") -> (.not. x?=w280:bool)
        n199 = case shown="True" "bypass Shunt" {
          tunnel: [T5."Turn Off bypass - On Shunt" ("Bypass Shunt") T5."Turn On bypass - Off Shunt" ("Bypass Shunt")] -> w284
          frame False {
            # "add Shunt"
          }
          frame True {
            # "No Shunt"
          }
        }
        n200 = property on="schematic" class="Bool (strict)"("Value"=w280) -> ()  [unwired: 2 in, 2 out]
        n201 = property on="Ext PW Vol Monitor" class="Bool (strict)"() -> ("Value"=w278:bool)  [unwired: 2 in, 2 out]
        n202 = property on="Range - Shunts" class="Enum (strict)"() -> ("Value"=w282:T1)  [unwired: 2 in, 2 out]
        n203 = local read "Task out"() -> (w281:refnum<k21>)
        n204 = local read "USB"() -> (w283:tag)
        n205 = call "UEvent_SET_BYPASS_SHUNT_OR_NOT.vi"("Task in"=w281, "Ext PW Vol Monitor"=w278, "USB"=w283, "Bypass Shunt"=w284, "Range_shunt"=w282) -> ("error out"=→"error out 3":errorcluster, "Task out"=w275:refnum<k21>)  [unwired: 5 in]
        n206 = local read "Measure"() -> (w277:bool)
        n207 = local write "Task out"(w275) -> ()
        n208 = case shown="False" w277 {
          tunnel: w275 -> [_ w286]
          tunnel: [refnum<k21> "Stop" ("Refnum out") w286] -> w276
          frame False {
          }
          frame True {
          }
        }
        n209 = local write "Task out"(w276) -> ()
      }
      event "Power ON/OFF": Value Change {
        n210 = event-data() -> ()  [unwired: 1 in, 6 out]
        n211 = case shown="False" "Power ON/OFF" {
          tunnel: [enum16{"Power ON DUT", "Power OFF DUT"}."Power OFF DUT" ("Power ON/OFF DUT") enum16{"Power ON DUT", "Power OFF DUT"}."Power ON DUT" ("Power ON/OFF DUT")] -> w298
          frame False {
          }
          frame True {
            # "ON"
          }
        }
        n212 = local read "Vout  - Vbat profile"() -> (w297:enum16{"3.8VDC", "2.9VDC", "By Pass", "4.0VDC"})
        n213 = property on="Ext PW Vol Monitor" class="Bool (strict)"() -> ("Value"=w293:bool)  [unwired: 2 in, 2 out]
        n214 = property on="Range - Shunts" class="Enum (strict)"() -> ("Value"=w296:T1)  [unwired: 2 in, 2 out]
        n215 = local read "Task out"() -> (w300:refnum<k21>)
        n216 = local read "USB"() -> (w295:tag)
        n217 = call "UEvent_ON_OFF_POWER_SOURCE.vi"("USB"=w295, "Power ON/OFF DUT"=w298, "Ext PW Vol Monitor"=w293, "Value"=w296, "Vout  - Vbat profile"=w297, "Refnum in"=w300) -> ("Battery_Voltage"=w299:dbl, "DUT_Voltage"=w289:dbl, "Refnum out"=w290:refnum<k21>)  [unwired: 3 in]
        n218 = local read "Measure"() -> (w292:bool)
        n219 = local write "PW_Internal_Source"(w299) -> ()
        n220 = local write "Vbat"(w289) -> ()
        n221 = local write "Task out"(w290) -> ()
        n222 = case shown="False" w292 {
          tunnel: w290 -> [_ w302]
          tunnel: [refnum<k21> "Stop" ("Refnum out") w302] -> w291
          frame False {
          }
          frame True {
          }
        }
        n223 = local write "Task out"(w291) -> ()
        n224 = local write "vbat_lb"(w289) -> ()
        "POWER ON_OFF" <- "Power ON/OFF"
      }
      event "Profile": Value Change {
        n225 = event-data() -> ()  [unwired: 1 in, 6 out]
        n226 = case shown="\"Hi-POWER\"" "Profile" {
          tunnel: [enum16{"3.8VDC", "2.9VDC", "By Pass", "4.0VDC"}."2.9VDC" ("DUT Voltage Selector") enum16{"3.8VDC", "2.9VDC", "By Pass", "4.0VDC"}."By Pass" ("DUT Voltage Selector") enum16{"3.8VDC", "2.9VDC", "By Pass", "4.0VDC"}."3.8VDC" ("DUT Voltage Selector") enum16{"3.8VDC", "2.9VDC", "By Pass", "4.0VDC"}."By Pass" ("DUT Voltage Selector")] -> w305
          frame "SAM", Default {
          }
          frame "Other..." {
          }
          frame "DIANA" {
          }
          frame "Hi-POWER" {
          }
        }
        n227 = local write "Vout  - Vbat profile"(w305) -> ()
      }
      event "Waveform_main": Cursor Move {
        n228 = event-data() -> ()  [unwired: 1 in, 9 out]
        n229 = local read "Waveform_main"() -> (w319:waveform(sgl))
        n230 = property on="Waveform_main" class="WFGraph (strict)"() -> ("CrsrList"=w329:T6)  [unwired: 2 in, 2 out]
        n231 = local read "Sample rate"() -> (w318:dbl)
        n232 = call "uA_daq_Capture_Current_waveform_to_new_chart.vi"("Sample rate"=w318, "CrsrList"=w329, "Waveform_main"=w319) -> ("Numeric"=w326:dbl, "Waveform"=w327:waveform(sgl), "Numeric 2"=w328:sgl)  [unwired: 6 in]
        n233 = local write "Avg"(w328) -> ()
        n234 = local write "Waveform_sub"(w327) -> ()
        n235 = property on="Waveform_sub" class="WFGraph (strict)"("XScale.Maximum"=w326, "XScale.Minimum"=0.0 ("X Scale.Range:Minimum")) -> (error out=w311:errorcluster)  [unwired: 2 in, 1 out]
        n236 = property on="Waveform_main" class="WFGraph (strict)"(error in=w311, "Active Cursor"=u32 1) -> (error out=w321:errorcluster, "Value"=w320:waveform(sgl), "Cursor.Cursor X"=w323:dbl)  [unwired: 1 in, 1 out]
        n237 = property on="Waveform_main" class="WFGraph (strict)" props=["CrsrList", "Active Cursor", "Cursor", "Cursor X"](error in=w321, "Active Cursor"=u32 0) -> ("Cursor.Cursor X"=w322:dbl)  [unwired: 1 in, 3 out]
        n238 = local read "Sample rate"() -> (w317:dbl)
        n239 = call "uA_daq_calculate_All_values_from Sub_chart.vi"("Cursor.Cursor X 2"=w323, "Cursor.Cursor X"=w322, "Value"=w320, "Sample rate"=w317) -> ("Max value"=→"Max":dbl, "Average"=→"Avg":dbl, "Delta(s)"=→"Delta(s)":sgl, "Min value"=→"Min":dbl)  [unwired: 4 in]
      }
      event "Calib": Value Change {
        n240 = event-data() -> ()  [unwired: 1 in, 6 out]
        n241 = case shown="False" FALSE {
          frame False {
            w344 = 3.0  # Coef 10Ohm:3
            # "uA"
            n242 = flat-sequence {
              tunnel: [w359] -> w342
              frame #0 {
                n243 = call "Display Message to User2"() -> ()  [unwired: 10 in, 2 out]
                n244 = local write "Measure"(FALSE ("Measure")) -> ()
              }
              frame #1 {
                n245 = local read "Task out"() -> (w356:refnum<k21>)
                n246 = Wait (ms)(milliseconds to wait=u32 1000) -> ()  [unwired: 1 out]
                n247 = call <vilib>:"DAQmx Stop Task.vi"("task/channels in"=w356) -> ("task out"=w355:refnum<k21>, "error out"=w357:errorcluster)  [unwired: 13 in]
                n248 = call <vilib>:"DAQmx Clear Task.vi"("task in"=w355, "error in"=w357) -> ("error out"=w354:errorcluster)  [unwired: 13 in]
                n249 = case shown="No Error" w354 {
                  frame No Error {
                    n250 = local write "Task out"(refnum<k21> "Stop" ("y")) -> ()
                  }
                  frame Error {
                  }
                }
                n251 = local read "USB"() -> (w359:tag)
              }
            }
            n252 = call "uA_daq_Set_ext_power_CM2_DIANA_LOG_Bat.vi"("USB DAQ in"=w342) -> ("error out"=w339:errorcluster, "USB DAQ out"=w346:tag)  [unwired: 9 in]
            n253 = call "uA__daq_Set_diana_uA_Vbat_for_reading.vi"("error in (no error)"=w339, "USB DAQ in"=w346) -> ("error out"=w340:errorcluster, "Refnum out"=w345:refnum<k21>)  [unwired: 8 in]
            n254 = for {
              N: 5 -> [_]
              tunnel: w345 -> [w352]
              tunnel: w344 -> [w351]
              tunnel: [w350] -> w343
              tunnel: [w347] -> w334 mode=indexing
              shift-right: [w349] -> w341
              shift-left: w340 -> [w348]
              n255 = call "uA__daq_Get_diana_uA_Vbat_for_reading.vi"("error in (no error)"=w348, "Coef"=w351, "Refnum in"=w352) -> ("error out"=w349:errorcluster, "uA Current"=w350:dbl, "mA_offsect"=w347:dbl)  [unwired: 3 in, 3 out]
            }
            n256 = Add Array Elements(numeric array=w334) -> (sum=w335:dbl)
            n257 = local write "uA_bank0"(w343) -> ()
            n258 = Array Size(array=w334) -> (size(s)=w336:i32)
            n259 = Divide(x=w335, y=w336) -> (x/y=w333:dbl)
            n260 = call "Calibration_Read_streaming_3s.vi"("error in (no error)"=w341, "USB"=w342) -> ("error out"=w332:errorcluster, "uABank1"=w338:dbl)  [unwired: 8 in]
            "uA_bank1" <- w338
            n261 = call "Display Message to User3"("error in (no error)"=w332, "Enable"=TRUE) -> ()  [unwired: 8 in, 2 out]
            n262 = local write "mARange"(w333) -> ()
            n263 = call "Calibration_Save_file.vi"("mA"=w333, "USB_DEV"=w342, "uABank1"=w338, "uABank0"=w343) -> ()  [unwired: 8 in]
          }
          frame True {
            # "mA"
          }
        }
      }
      event "Clear Graph": Value Change {
        n264 = event-data() -> ()  [unwired: 1 in, 6 out]
        n265 = flat-sequence {
          frame #0 {
            w361 = waveform(sgl) {"t0"=timestamp(0 s since 1904-01-01), "dt"=1.0, "Y"=[]} ("Waveform_main")
            n266 = local write "Clear"(TRUE ("Clear")) -> ()
            n267 = Wait (ms)(milliseconds to wait=u32 500) -> ()  [unwired: 1 out]
            n268 = local write "Waveform_main"(w361) -> ()
            n269 = local write "Waveform_sub"(w361) -> ()
          }
          frame #1 {
            n270 = local write "Clear"(FALSE ("Clear")) -> ()
          }
        }
      }
      event "ZOOM +": Value Change {
        n271 = event-data() -> ()  [unwired: 1 in, 6 out]
        n272 = property on="Waveform_main" class="WFGraph (strict)" props=["XScale", "Range", "XScale", "Increment", "XScale", "Maximum", "XScale", "Minimum"]() -> ("XScale.Maximum"=w370:dbl, "XScale.Minimum"=w366:dbl)  [unwired: 2 in, 4 out]
        n273 = Subtract(x=w370, y=0.1) -> (x-y=w368:dbl)
        n274 = Add(x=w366, y=0.1) -> (x+y=w365:dbl)
        n275 = property on="Waveform_main" class="WFGraph (strict)"("XScale.Maximum"=w368, "XScale.Minimum"=w365) -> ()  [unwired: 2 in, 2 out]
      }
      event "ZOOM -": Value Change {
        n276 = event-data() -> ()  [unwired: 1 in, 6 out]
        n277 = property on="Waveform_main" class="WFGraph (strict)" props=["XScale", "Range", "XScale", "Increment", "XScale", "Maximum", "XScale", "Minimum"]() -> ("XScale.Maximum"=w379:dbl, "XScale.Minimum"=w375:dbl)  [unwired: 2 in, 4 out]
        n278 = Subtract(x=w375, y=0.1) -> (x-y=w372:dbl)
        n279 = Less Than 0?(x=w372) -> (x < 0?=w374:bool)
        n280 = Add(x=w379, y=0.1) -> (x+y=w377:dbl)
        n281 = Select(t=0.0, s=w374, f=w372) -> (s? t:f=w371:dbl)
        n282 = property on="Waveform_main" class="WFGraph (strict)"("XScale.Maximum"=w377, "XScale.Minimum"=w371) -> ()  [unwired: 2 in, 2 out]
      }
      event "ZOOM M1M2": Value Change {
        n283 = event-data() -> ()  [unwired: 1 in, 6 out]
        n284 = property on="Waveform_main" class="WFGraph (strict)"("Active Cursor"=u32 0) -> (error out=w386:errorcluster)  [unwired: 2 in, 1 out]
        n285 = property on="Waveform_main" class="WFGraph (strict)"(error in=w386) -> (error out=w383:errorcluster, "Cursor.Cursor X"=w381:dbl)  [unwired: 1 in, 1 out]
        n286 = property on="Waveform_main" class="WFGraph (strict)"(error in=w383, "Active Cursor"=u32 1) -> (error out=w385:errorcluster)  [unwired: 1 in, 1 out]
        n287 = property on="Waveform_main" class="WFGraph (strict)"(error in=w385) -> ("Cursor.Cursor X"=w380:dbl)  [unwired: 1 in, 2 out]
        n288 = Greater?(x=w381, y=w380) -> (0:w382:bool)
        n289 = case shown="True" w382 {
          tunnel: w381 -> [w389 w391]
          tunnel: w380 -> [w388 w390]
          frame False {
            n290 = property on="Waveform_main" class="WFGraph (strict)"("XScale.Maximum"=w388, "XScale.Minimum"=w389) -> ()  [unwired: 2 in, 2 out]
          }
          frame True {
            n291 = property on="Waveform_main" class="WFGraph (strict)"("XScale.Maximum"=w391, "XScale.Minimum"=w390) -> ()  [unwired: 2 in, 2 out]
          }
        }
      }
      event "Waveform_main": Mouse Down {
        n292 = event-data() -> ()  [unwired: 1 in, 8 out]
      }
      event "Tab Control": Value Change {
        n293 = event-data() -> ()  [unwired: 1 in, 6 out]
      }
      event "Center": Value Change {
        n294 = event-data() -> ()  [unwired: 1 in, 6 out]
        n295 = property on="Waveform_main" class="WFGraph (strict)"() -> ("XScale.Maximum"=w396:dbl, "XScale.Minimum"=w395:dbl)  [unwired: 2 in, 2 out]
        n296 = Add(x=w396, y=w395) -> (x+y=w394:dbl)
        n297 = Divide(x=w394, y=2.0) -> (x/y=w392:dbl)
        n298 = property on="Waveform_main" class="WFGraph (strict)" props=["Value", "Active Cursor", "Cursor", "Cursor X"]("Active Cursor"=u32 1, "Cursor.Cursor X"=w392) -> (error out=w397:errorcluster)  [unwired: 2 in, 2 out]
        n299 = property on="Waveform_main" class="WFGraph (strict)" props=["CrsrList", "Active Cursor", "Cursor", "Cursor X"](error in=w397, "Active Cursor"=u32 0, "Cursor.Cursor X"=w392) -> ()  [unwired: 1 in, 3 out]
      }
      event "stop": Value Change {
        n300 = event-data() -> ()  [unwired: 1 in, 6 out]
        n301 = flat-sequence {
          tunnel: [w404] -> w400
          tunnel: w400 -> [w413]
          frame #0 {
            n302 = local write "Task out"(refnum<k21> "Stop" ("Task out")) -> ()
          }
          frame #1 {
            n303 = local read "USB"() -> (w412:tag)
            n304 = local read "Task out"() -> (w407:refnum<k21>)
            n305 = call "uA_daq_Set_Relay_internal_power_on_off_from_baterry.vi"("Power ON/OFF DUT"=enum16{"Power ON DUT", "Power OFF DUT"}."Power OFF DUT", "USB DAQ"=w412) -> ("error out"=w403:errorcluster)  [unwired: 9 in]
            n306 = local read "USB"() -> (w410:tag)
            n307 = call <vilib>:"DAQmx Stop Task.vi"("task/channels in"=w407, "error in"=w403) -> ("task out"=w402:refnum<k21>, "error out"=w405:errorcluster)  [unwired: 12 in]
            n308 = call <vilib>:"DAQmx Clear Task.vi"("task in"=w402, "error in"=w405) -> ("error out"=w406:errorcluster)  [unwired: 13 in]
            n309 = call <vilib>:"Clear Errors.vi"("error in (no error)"=w406) -> ("error out"=w409:errorcluster)  [unwired: 5 in, 1 out]
            n310 = call "uA_daq_ON_OFF_LED_Measure.vi"("error in"=w409, "LED_meas"=FALSE ("Boolean"), "USB"=w410) -> ("error out"=w404:errorcluster)  [unwired: 8 in]
          }
          frame #2 {
            n311 = call <vilib>:"Clear Errors.vi"("error in (no error)"=w413) -> ()  [unwired: 5 in, 2 out]
            n312 = local read "Ver"() -> (w414:string)
            n313 = Empty String/Path?(string/path=w414) -> (empty?=w415:bool)
            n314 = case shown="False" w415 {
              frame True {
              }
              frame False {
                n315 = Quit LabVIEW(quit? (T)=TRUE) -> ()
              }
            }
          }
          frame #3 {
            n316 = Stop(stop? (T)=TRUE) -> ()
          }
        }
      }
      event "Save": Value Change {
        n317 = event-data() -> ()  [unwired: 1 in, 6 out]
        n318 = local read "Waveform_main"() -> (w419:waveform(sgl))
        n319 = call "File Dialog"("pattern (all files)"="*.dlog", "pattern label"="datalog") -> ("selected path"=w422:path)  [unwired: 10 in, 3 out]
        n320 = call-poly <vilib>:"Write Waveforms to File.vi"("append to file? (new file:F)"=FALSE, "waveform"=w419, "file path (dialog if empty)"=w422) -> ()  [unwired: 7 in, 2 out]
      }
      event "Load": Value Change {
        (unwired) FALSE ("append to file? (new file:F)")
        n321 = event-data() -> ()  [unwired: 1 in, 6 out]
        n322 = call "File Dialog3"("pattern (all files)"="*.dlog", "pattern label"="datalog") -> ("selected path"=w426:path)  [unwired: 10 in, 3 out]
        n323 = call-poly <vilib>:"Read Waveforms from File.vi"("file path (dialog if empty)"=w426) -> ("first waveform in record"=w423:waveform(dbl))  [unwired: 5 in, 3 out]
        n324 = local write "Waveform_main"(w423) -> ()
      }
      event "Take Picture": Value Change {
        n325 = event-data() -> ()  [unwired: 1 in, 6 out]
        n326 = call <vilib>:"Application Directory.vi"() -> ("Application Directory"=w428:path)
        n327 = call "File Dialog2"("start path"=w428, "pattern (all files)"="*.jpg", "pattern label"="*.jpg") -> ("selected path"=w434:path, "error out"=w431:errorcluster)  [unwired: 9 in, 2 out]
        n328 = control-ref of="This VI"() -> (w432:refnum<vi>)
        n329 = invoke on="Invoke Node" class="VI" method="FP.Get Image"(reference=w432, "image depth"=enum32{"File", "Clipboard"}."File" ("Target")) -> ("image data"=w433:T7)  [unwired: 4 in, 5 out]
        n330 = call <vilib>:"Clear Errors.vi"("error in (no error)"=w431) -> ()  [unwired: 5 in, 2 out]
        n331 = call <vilib>:"Write JPEG File.vi"("image data"=w433, "path to JPEG file"=w434) -> ()  [unwired: 8 in, 2 out]
      }
      event "Save setting": Value Change {
        w456 = "SETTING" ("section")
        n332 = event-data() -> ()  [unwired: 1 in, 6 out]
        n333 = call <vilib>:"Application Directory.vi"() -> ("Application Directory"=w461:path)
        n334 = Build Path(base path=w461, name or relative path="Setting.cfg") -> (appended path=w459:path)
        n335 = local read "Range - Shunts"() -> (w449:T1)
        n336 = call <vilib>:"Open Config Data.vi"("create file if necessary (T)"=TRUE, "configuration file path"=w459) -> ("error out"=w435:errorcluster, "refnum"=w457:T3)  [unwired: 7 in, 1 out]
        n337 = local read "Profile"() -> (w448:enum16{"SAM", "DIANA", "Hi-POWER", "Other..."})
        n338 = local read "Vout  - Vbat profile"() -> (w446:enum16{"3.8VDC", "2.9VDC", "By Pass", "4.0VDC"})
        n339 = call-poly <vilib>:"Write Key.vi"("section"=w456, "error in (no error)"=w435, "value"=w449, "key"="Range - Shunts", "refnum"=w457) -> ("error out"=w436:errorcluster, "refnum out"=w454:T3)  [unwired: 4 in, 1 out]
        n340 = call-poly <vilib>:"Write Key.vi"("section"=w456, "error in (no error)"=w436, "value"=w448, "key"="Profile", "refnum"=w454) -> ("error out"=w437:errorcluster, "refnum out"=w455:T3)  [unwired: 4 in, 1 out]
        n341 = local read "Internal PW"() -> (w444:bool)
        n342 = call-poly <vilib>:"Write Key.vi"("section"=w456, "error in (no error)"=w437, "value"=w446, "key"="Vout  - Vbat profile", "refnum"=w455) -> ("error out"=w438:errorcluster, "refnum out"=w453:T3)  [unwired: 4 in, 1 out]
        n343 = local read "bypass Shunt"() -> (w442:bool)
        n344 = call-poly <vilib>:"Write Key.vi"("section"=w456, "error in (no error)"=w438, "value"=w444, "key"="Internal PW", "refnum"=w453) -> ("error out"=w439:errorcluster, "refnum out"=w452:T3)  [unwired: 4 in, 1 out]
        n345 = call-poly <vilib>:"Write Key.vi"("section"=w456, "error in (no error)"=w439, "value"=w442, "key"="bypass Shunt", "refnum"=w452) -> ("error out"=w440:errorcluster, "refnum out"=w441:T3)  [unwired: 4 in, 1 out]
        n346 = call <vilib>:"Close Config Data.vi"("error in (no error)"=w440, "refnum"=w441) -> ()  [unwired: 8 in, 2 out]
      }
    }
  }
  n347 = while {
    tunnel: w2 -> [w470]
    tunnel: [w469] -> w11
    shift-right: [w465] -> w4
    shift-left: w3 -> [w467]
    stop <- FALSE ("stop (F)") stop-if-true
    n348 = local read "Range - Shunts"() -> (w464:T1)
    n349 = Equal?(x=w467, y=refnum<k21> "Stop") -> (x = y?=w463:bool)
    n350 = case shown="False" w463 {
      tunnel: w470 -> [w473 w480]
      tunnel: [w473 w479] -> w469
      tunnel: w467 -> [_ w476]
      tunnel: [w472 w478] -> w465
      tunnel: w464 -> [_ w477]
      tunnel: refnum<k21> refnum ("task out") -> [_ w474]
      frame True {
        n351 = local read "Task out"() -> (w472:refnum<k21>)
        n352 = Wait (ms)(milliseconds to wait=u32 100) -> ()  [unwired: 1 out]
      }
      frame False {
        n353 = Not Equal?(x=w476, y=w474) -> (x != y?=w475:bool)
        n354 = case shown="True" w475 {
          tunnel: w480 -> [w482 w487]
          tunnel: [w482 w486] -> w479
          tunnel: w476 -> [_ w485]
          tunnel: [w481 w484] -> w478
          tunnel: w477 -> [_ w483]
          frame False {
            n355 = local read "Task out"() -> (w481:refnum<k21>)
          }
          frame True {
            n356 = case shown="\"mA Range Rs = 1ohm\"" w483 {
              tunnel: w487 -> [w493 w503 w513 w523]
              tunnel: [w492 w502 w512 w522] -> w486
              tunnel: w485 -> [w491 w501 w511 w521]
              tunnel: [w490 w500 w510 w520] -> w484
              frame "mA Range Rs = 1ohm" {
                n357 = call "DAQ_ADC_Max_Sample_Rate_For_USB_6001.vi"("Refnum in"=w491) -> ("error out"=w489:errorcluster, "data"=w488:waveform(dbl))  [unwired: 9 in]
                n358 = case shown="No Error" w489 {
                  selector: w489 -> [_ w497]
                  tunnel: w493 -> [w496 _]
                  tunnel: [w495 _] -> w492
                  tunnel: w488 -> [w494 _]
                  frame No Error {
                    n359 = Enqueue Element(queue=w496, element=w494) -> (queue out=w495:refnum<queue>)  [unwired: 2 in, 2 out]
                  }
                  frame Error {
                    n360 = call <vilib>:"Clear Errors.vi"("error in (no error)"=w497) -> ()  [unwired: 5 in, 2 out]
                  }
                }
                n361 = local read "Task out"() -> (w490:refnum<k21>)
              }
              frame "mA Range Rs = 1ohm - X2" {
                n362 = call "DAQ_ADC_Max_Sample_Rate_For_USB_6001.vi"("Refnum in"=w501) -> ("error out"=w499:errorcluster, "data"=w498:waveform(dbl))  [unwired: 9 in]
                n363 = case shown="No Error" w499 {
                  selector: w499 -> [_ w507]
                  tunnel: w503 -> [w506 _]
                  tunnel: [w505 _] -> w502
                  tunnel: w498 -> [w504 _]
                  frame No Error {
                    n364 = Enqueue Element(queue=w506, element=w504) -> (queue out=w505:refnum<queue>)  [unwired: 2 in, 2 out]
                  }
                  frame Error {
                    n365 = call <vilib>:"Clear Errors.vi"("error in (no error)"=w507) -> ()  [unwired: 5 in, 2 out]
                  }
                }
                n366 = local read "Task out"() -> (w500:refnum<k21>)
              }
              frame "mA Range Rs = 3.3ohm" {
                n367 = call "DAQ_ADC_Max_Sample_Rate_For_USB_6001.vi"("Refnum in"=w511) -> ("error out"=w509:errorcluster, "data"=w508:waveform(dbl))  [unwired: 9 in]
                n368 = case shown="No Error" w509 {
                  selector: w509 -> [_ w517]
                  tunnel: w513 -> [w516 _]
                  tunnel: [w515 _] -> w512
                  tunnel: w508 -> [w514 _]
                  frame No Error {
                    n369 = Enqueue Element(queue=w516, element=w514) -> (queue out=w515:refnum<queue>)  [unwired: 2 in, 2 out]
                  }
                  frame Error {
                    n370 = call <vilib>:"Clear Errors.vi"("error in (no error)"=w517) -> ()  [unwired: 5 in, 2 out]
                  }
                }
                n371 = local read "Task out"() -> (w510:refnum<k21>)
              }
              frame "uA Range  Rs = 3.3ohm" {
                n372 = call "DAQ_ADC_Max_Sample_Rate_For_USB_6001.vi"("Refnum in"=w521) -> ("error out"=w519:errorcluster, "data"=w518:waveform(dbl))  [unwired: 9 in]
                n373 = local read "Task out"() -> (w520:refnum<k21>)
                n374 = case shown="No Error" w519 {
                  selector: w519 -> [_ w527]
                  tunnel: w523 -> [w526 _]
                  tunnel: [w525 _] -> w522
                  tunnel: w518 -> [w524 _]
                  frame No Error {
                    n375 = Enqueue Element(queue=w526, element=w524) -> (queue out=w525:refnum<queue>)  [unwired: 2 in, 2 out]
                  }
                  frame Error {
                    n376 = call <vilib>:"Clear Errors.vi"("error in (no error)"=w527) -> ()  [unwired: 5 in, 2 out]
                  }
                }
              }
            }
          }
        }
      }
    }
  }
  n377 = while {
    tunnel: w2 -> [w540]
    stop <- FALSE stop-if-true
    w535 = 24164516  # 1200s
    n378 = property on="Range - Shunts" class="Enum (strict)"() -> ("Value"=w530:T1)  [unwired: 2 in, 2 out]
    n379 = disable-structure shown="Enabled" {
      disable-tunnel: _ -> [w576 _]
      disable-tunnel: [w575 _] -> _
      frame Disabled {
        n380 = call "Compensation_mA_100mA_Peaks.vi"("Waveform in"=w576) -> ("Waveform out"=w575:waveform(sgl))  [unwired: 10 in]
      }
      frame Enabled {
      }
    }
    n381 = property on="Ext PW Vol Monitor" class="Bool (strict)"() -> ("Value"=w533:bool)  [unwired: 2 in, 2 out]
    n382 = local read "Clear"() -> (w539:bool)
    n383 = Dequeue Element(queue=w540) -> (element=w531:waveform(sgl))  [unwired: 2 in, 3 out]
    n384 = case shown="\"uA Range  Rs = 3.3ohm\"" w530 {
      tunnel: w531 -> [w546 w550 w554 w558]
      tunnel: [w543 w547 w551 w555] -> w529
      frame "mA Range Rs = 3.3ohm" {
        n385 = call-poly <vilib>:"Basic Averaged DC-RMS.vi"("signal in"=w546) -> ("RMS value"=w544:dbl)  [unwired: 7 in, 3 out]
        n386 = Greater?(x=w544, y=3.5) -> (0:w543:bool)
      }
      frame "uA Range  Rs = 3.3ohm" {
        n387 = call-poly <vilib>:"Basic Averaged DC-RMS.vi"("signal in"=w550) -> ("RMS value"=w548:dbl)  [unwired: 7 in, 3 out]
        n388 = Greater?(x=w548, y=3.5) -> (0:w547:bool)
      }
      frame "mA Range Rs = 1ohm" {
        n389 = call-poly <vilib>:"Basic Averaged DC-RMS.vi"("signal in"=w554) -> ("RMS value"=w552:dbl)  [unwired: 7 in, 3 out]
        n390 = Greater?(x=w552, y=2.0) -> (0:w551:bool)
      }
      frame "mA Range Rs = 1ohm - X2" {
        n391 = call-poly <vilib>:"Basic Averaged DC-RMS.vi"("signal in"=w558) -> ("RMS value"=w556:dbl)  [unwired: 7 in, 3 out]
        n392 = Greater?(x=w556, y=2.0) -> (0:w555:bool)
      }
    }
    n393 = case shown="True" w533 {
      tunnel: w531 -> [w566 w574]
      tunnel: [w566 w572] -> w534
      tunnel: w529 -> [_ w570]
      tunnel: [FALSE w570] -> w528
      frame True {
        n394 = Unbundle By Name(w566) -> ("Y"=w565:sgl[])
        n395 = Add Array Elements(numeric array=w566) -> (sum=w563:sgl)
        n396 = Array Size(array=w565) -> (size(s)=w564:i32)
        n397 = Divide(x=w563, y=w564) -> (x/y=w560:sgl)
        n398 = Greater?(x=w560, y=6) -> (0:w562:bool)
        n399 = case shown="True" w562 {
          frame False {
          }
          frame True {
            n400 = property on="Internal PW" class="Bool (strict)"("Value"=FALSE ("Internal PW")) -> ()  [unwired: 2 in, 2 out]
            n401 = local read "USB"() -> (w569:tag)
            n402 = call "uA_daq_switch_external_internal_pw_source.vi"("USB DAQ"=w569, "Ex/Int PW"=T4."Internal PW Source") -> ()  [unwired: 9 in, 1 out]
          }
        }
      }
      frame False {
        n403 = property on="Range - Shunts" class="Enum (strict)"() -> ("Value"=w571:T1)  [unwired: 2 in, 2 out]
        n404 = local read "mARange"() -> (w573:dbl)
        n405 = call "uA_daq_gain_caculator.vi"("Waveform Chart in"=w574, "Calib_value"=w573, "Range - Shunts"=w571) -> ("Waveform out"=w572:waveform(dbl))  [unwired: 12 in]
      }
    }
    n406 = case shown="False" w539 {
      tunnel: [waveform(sgl) {"t0"=timestamp(0 s since 1904-01-01), "dt"=1.0, "Y"=[]} ("Waveform_main") w592] -> w538
      frame True {
      }
      frame False {
        n407 = local read "Waveform_main"() -> (w592:waveform(sgl))
      }
    }
    n408 = property on="out_range" class="Bool (strict)"("Visible"=w528) -> ()  [unwired: 2 in, 2 out]
    n409 = Unbundle By Name(w538) -> ("Y"=w532:sgl[])
    n410 = local read "Measure"() -> (w537:bool)
    n411 = Array Size(array=w532) -> (size(s)=w541:i32)
    n412 = Greater Or Equal?(x=w541, y=w535) -> (x >= y?=w536:bool)
    n413 = case shown="False" w536 {
      tunnel: w534 -> [_ w581]
      tunnel: w538 -> [_ w580]
      tunnel: w537 -> [w577 w579]
      frame True {
        n414 = local write "Measure"(FALSE ("Measure")) -> ()
        n415 = case shown="True" w577 {
          frame False {
          }
          frame True {
            n416 = call "Display Message to User4"() -> ()  [unwired: 10 in, 2 out]
          }
        }
      }
      frame False {
        n417 = case shown="True" w579 {
          tunnel: w581 -> [_ w589]
          tunnel: w580 -> [_ w583]
          frame False {
          }
          frame True {
            n418 = Subtract(x=w589, y=sgl 0.0) -> (x-y=w584:waveform(dbl))
            n419 = local read "Waveform_main"() -> (w586:waveform(sgl))
            n420 = call "WDT Append Waveforms SGL.vi"("waveform B"=w583, "waveform A"=w584) -> ("waveform out"=→"Waveform_main":waveform(sgl))  [unwired: 8 in, 1 out]
            n421 = property on="Waveform_main" class="WFGraph (strict)"() -> ("CrsrList"=w587:T6)  [unwired: 2 in, 2 out]
            n422 = local read "Sample rate"() -> (w585:dbl)
            n423 = call "uA_daq_capture_small_curr_waveform.vi"("Sample rate"=w585, "CrsrList"=w587, "Waveform_main"=w586) -> ("Numeric"=→"Average (uA)":sgl)  [unwired: 8 in]
          }
        }
      }
    }
  }
  n424 = Release Queue(queue=w11) -> ()  [unwired: 2 in, 3 out]
  n425 = call <vilib>:"DAQmx Clear Task.vi"("task in"=w4) -> ()  [unwired: 14 in, 1 out]
